vi "ex_SetAllExpressAttribs.vi"(7 "Enable (T if empty)":bool[](array[boolean]), 8 "error in":errorcluster, 9 "All Express Wave Attributes":T1[](array[typedef]) {"Timestamp" format="%<%X\n%x>T"; "Start Timestamp" format="%<%X\n%x>T"}, 11 "Signals":waveform(dbl)[](array[waveform])) -> (0 "error out":errorcluster, 3 "Signals With Attributes":waveform(dbl)[](array[waveform]))   [LabVIEW 2020]
uses:
  ex_WaveformAttribs.ctl
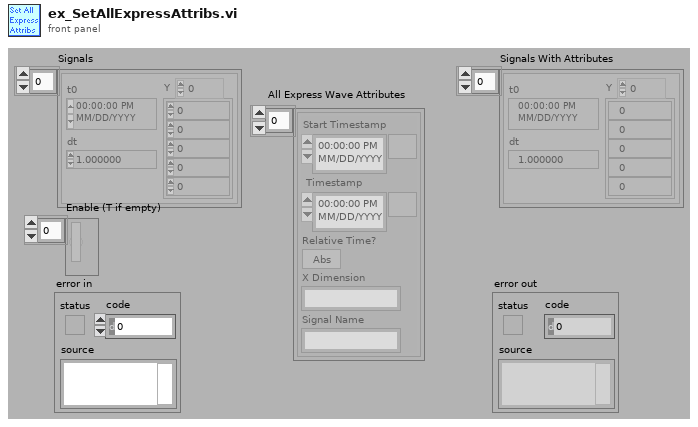
[diagram p1: front panel]
types:
  T1 = typedef "ex_WaveformAttribs.ctl" = cluster{"Start Timestamp":timestamp, "Timestamp":timestamp, "Relative Time?":bool, "X Dimension":string, "Signal Name":string}
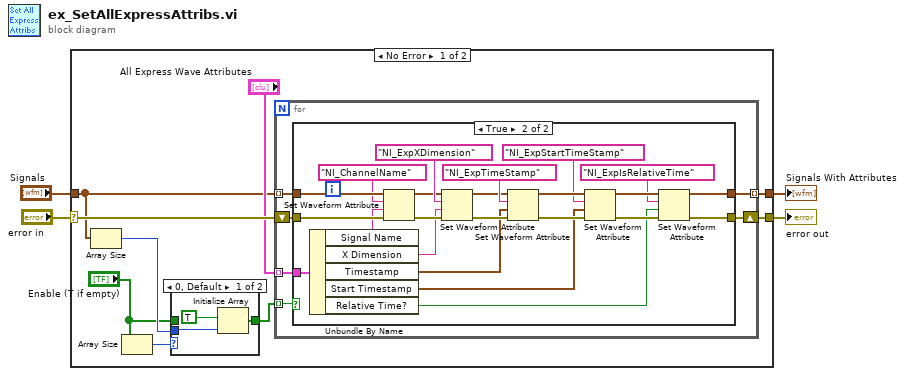
[diagram p0: block diagram]
diagram:
  n1 = case shown="No Error" "error in" {
    selector: "error in" -> [w11 w49]
    tunnel: [w13 w49] -> w4
    tunnel: [w12 w50] -> w1
    tunnel: "Signals" -> [w9 w50]
    frame No Error {
      n2 = Array Size(array=w9) -> (size(s)=w8:i32)
      n3 = Array Size(array="Enable (T if empty)") -> (size(s)=w5:i32)
      n4 = case shown="0, Default" w5 {
        tunnel: w8 -> [w15 _]
        tunnel: [w14 w17] -> w7
        tunnel: "Enable (T if empty)" -> [_ w17]
        frame 0, Default {
          n5 = Initialize Array(TRUE, w15) -> (w14:bool[])
        }
        frame 1.. {
        }
      }
      n6 = for {
        tunnel: w9 -> [w22] mode=indexing
        tunnel: [w19] -> w12 mode=indexing
        shift-right: [w23] -> w13
        shift-left: w11 -> [w21]
        tunnel: "All Express Wave Attributes" -> [w20] mode=indexing
        tunnel: w7 -> [w18] mode=indexing
        n7 = case shown="True" w18 {
          tunnel: [w24 w40] -> w23
          tunnel: w22 -> [w25 w39]
          tunnel: w21 -> [w24 w38]
          tunnel: w20 -> [_ w34]
          tunnel: [w25 w29] -> w19
          frame False {
          }
          frame True {
            n8 = Unbundle By Name(w34) -> ("Signal Name"=w28:string, "X Dimension"=w27:string, "Timestamp"=w26:timestamp, "Start Timestamp"=w31:timestamp, "Relative Time?"=w30:bool)
            n9 = Set Waveform Attribute(4:w38, 5:w28, 6:"NI_ChannelName" ("name"), 7:w39) -> (0:w35:errorcluster, 3:w36:waveform(dbl))  [unwired: 1 out]
            n10 = Set Waveform Attribute(4:w35, 5:w27, 6:"NI_ExpXDimension" ("name"), 7:w36) -> (0:w32:errorcluster, 3:w33:waveform(dbl))  [unwired: 1 out]
            n11 = Set Waveform Attribute(4:w32, 5:w26, 6:"NI_ExpTimeStamp" ("name"), 7:w33) -> (0:w44:errorcluster, 3:w45:waveform(dbl))  [unwired: 1 out]
            n12 = Set Waveform Attribute(4:w44, 5:w31, 6:"NI_ExpStartTimeStamp" ("name"), 7:w45) -> (0:w47:errorcluster, 3:w48:waveform(dbl))  [unwired: 1 out]
            n13 = Set Waveform Attribute(4:w47, 5:w30, 6:"NI_ExpIsRelativeTime" ("name"), 7:w48) -> (0:w40:errorcluster, 3:w29:waveform(dbl))  [unwired: 1 out]
          }
        }
      }
    }
    frame Error {
    }
  }
  "error out" <- w4
  "Signals With Attributes" <- w1
